vi "MiniCyc_Controller.vi"() -> ()   [LabVIEW 2024]
uses:
  <vilib>/Utility/file.llb/Write Delimited Spreadsheet (string).vi
panel:
  in  "Tab Control":T1(tab)
  in  "Tension Arc":dbl
  in  "Courant Arc":dbl
  in  "Réglage Arc :":enum32{"Item 0", "Item 1"}(radio)
  out "Tension effective Arc":dbl
  out "Courant effectif Arc":dbl
  in  "Courant Filament":dbl
  out "Courant effectif\nFilament":dbl
  in  "Débit Gaz m³/h":dbl(knob) scale=0.01..10.0 scale format="%#.6f"
  in  "Tension inflecteur":dbl min=0.0
  out "Tension I électrode 1":dbl
  out "Tension I électrode 2":dbl=-0.0
  out "Q2 Tension 2":dbl=-0.0
  in  "Tension quadrupole 2":dbl
  out "Q2 Tension 1":dbl
  out "Q1 Tension 2":dbl=-0.0
  in  "Tension quadrupole 1":dbl
  out "Q1 Tension 1":dbl
  in  "Tension Buncher":dbl
  out "Courant":bool=TRUE
  out "Débit Argon m³/h":dbl(knob) scale=0.0..10.0
  in  "Tension déflecteur":dbl min=0.0
  out "Tension D électrode 1":dbl
  out "Tension D électrode 2":dbl=-0.0
  in  "Tension Einzel":dbl
  in  "Tension Puller":dbl
  out "Tension effective\nEinzel":dbl
  out "Tension effective\nPuller":dbl
  out "Courant effectif\nBobine":dbl
  in  "Courant Bobine":dbl
  in  "Position\nPiston d'accord":dbl(knob) scale=0.01..10.0 scale format="%#.6f"
  out "Tension Crête":dbl
  out "Position effective\nPiston d'accord":dbl(slide) caption="Piston d'accord" scale=0.0..10.0
  in  "Amplificateur":dbl
  in  "Cible 1":enum32{"Item 0", "Item 1", "Radio Selection 3"}(radio)
  out "Courant Stripper1 Cible1":dbl
  out "Courant Stripper2 Cible1":dbl
  out "Courant Stripper3 Cible1":dbl
  in  "Rayon canne\nCible 1":dbl
  in  "Cible 2":enum32{"Item 0", "Item 1", "Radio Selection 3"}(radio)
  out "Courant Stripper1 Cible2":dbl
  out "Courant Stripper2 Cible2":dbl
  out "Courant Stripper3 Cible2":dbl
  in  "Rayon canne\nCible 2":dbl
  in  "Statut de la pompe":bool=TRUE
  out "Sonde 2 mbar":dbl(knob) scale=0.0..10.0
  out "Sonde 1 mbar":dbl(knob) scale=0.0..10.0
  out "Sonde 2 mbar":dbl(knob) scale=0.0..10.0
  out "Sonde 1 mbar":dbl(knob) scale=0.0..10.0
  out "Débit Eau\nBobine m³/h":dbl(knob) scale=0.0..10.0
  out "Débit Eau\nInflecteur m³/h":dbl(knob) scale=0.0..10.0
  out "Débit Eau\nDéflecteur m³/h":dbl(knob) scale=0.0..10.0
  out "Débit Eau\nLEBT m³/h":dbl(knob) scale=0.0..10.0
  out "Débit Eau\nSource m³/h":dbl(knob) scale=0.0..10.0
  out "Chemin du dossier":path
  in  "Limite de taille par fichiers":dbl=15.0
  in  "Activer l'enregistrement des données":bool=TRUE
  in  "Fréquence d'enregistrement des données":dbl=5.0
  # "KV"
  # "KV"
  # "mA"
  # "mA"
  # "µA"
  # "µA"
  # "KV"
  # "KV"
  # "KV"
  # "KV"
  # "KV"
  # "KV"
  # "KV"
  # "KV"
  # "KV"
  # "KV"
  # "KV"
  # "KV"
  # "KV"
  # "KV"
  # "KV"
  # "KV"
  # "KV"
  # "µA"
  # "µA"
  # "KV"
  # "µA"
  # "µA"
  # "µA"
  # "µA"
  # "µA"
  # "µA"
  # "Sec"
  # "Mb"
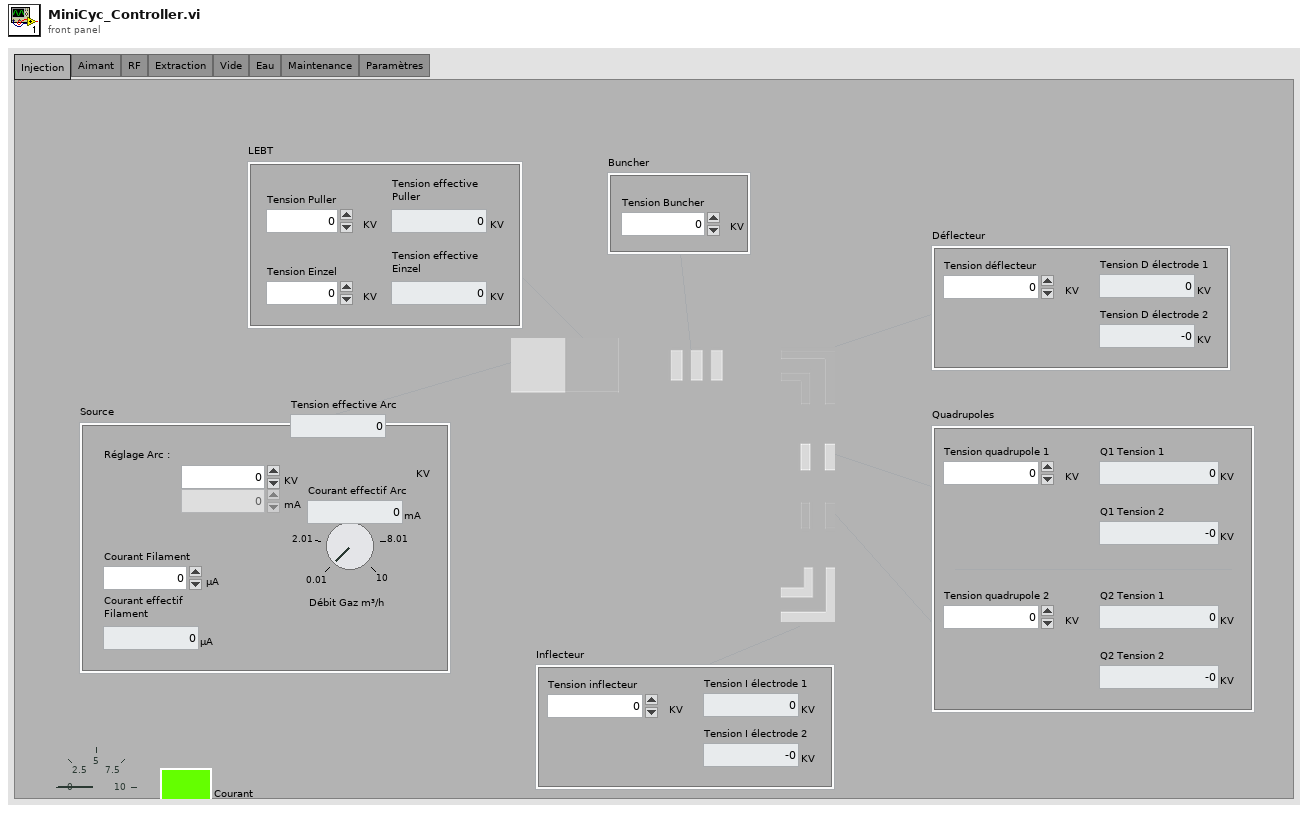
[diagram p1: front panel]
types:
  T1 = enum32{"Injection", "Aimant", "RF", "Extraction", "Vide", "Eau", "Maintenance", "Paramètres"}
  T2 = enum8{"Enabled", "Disabled", "Disabled and Grayed Out"}
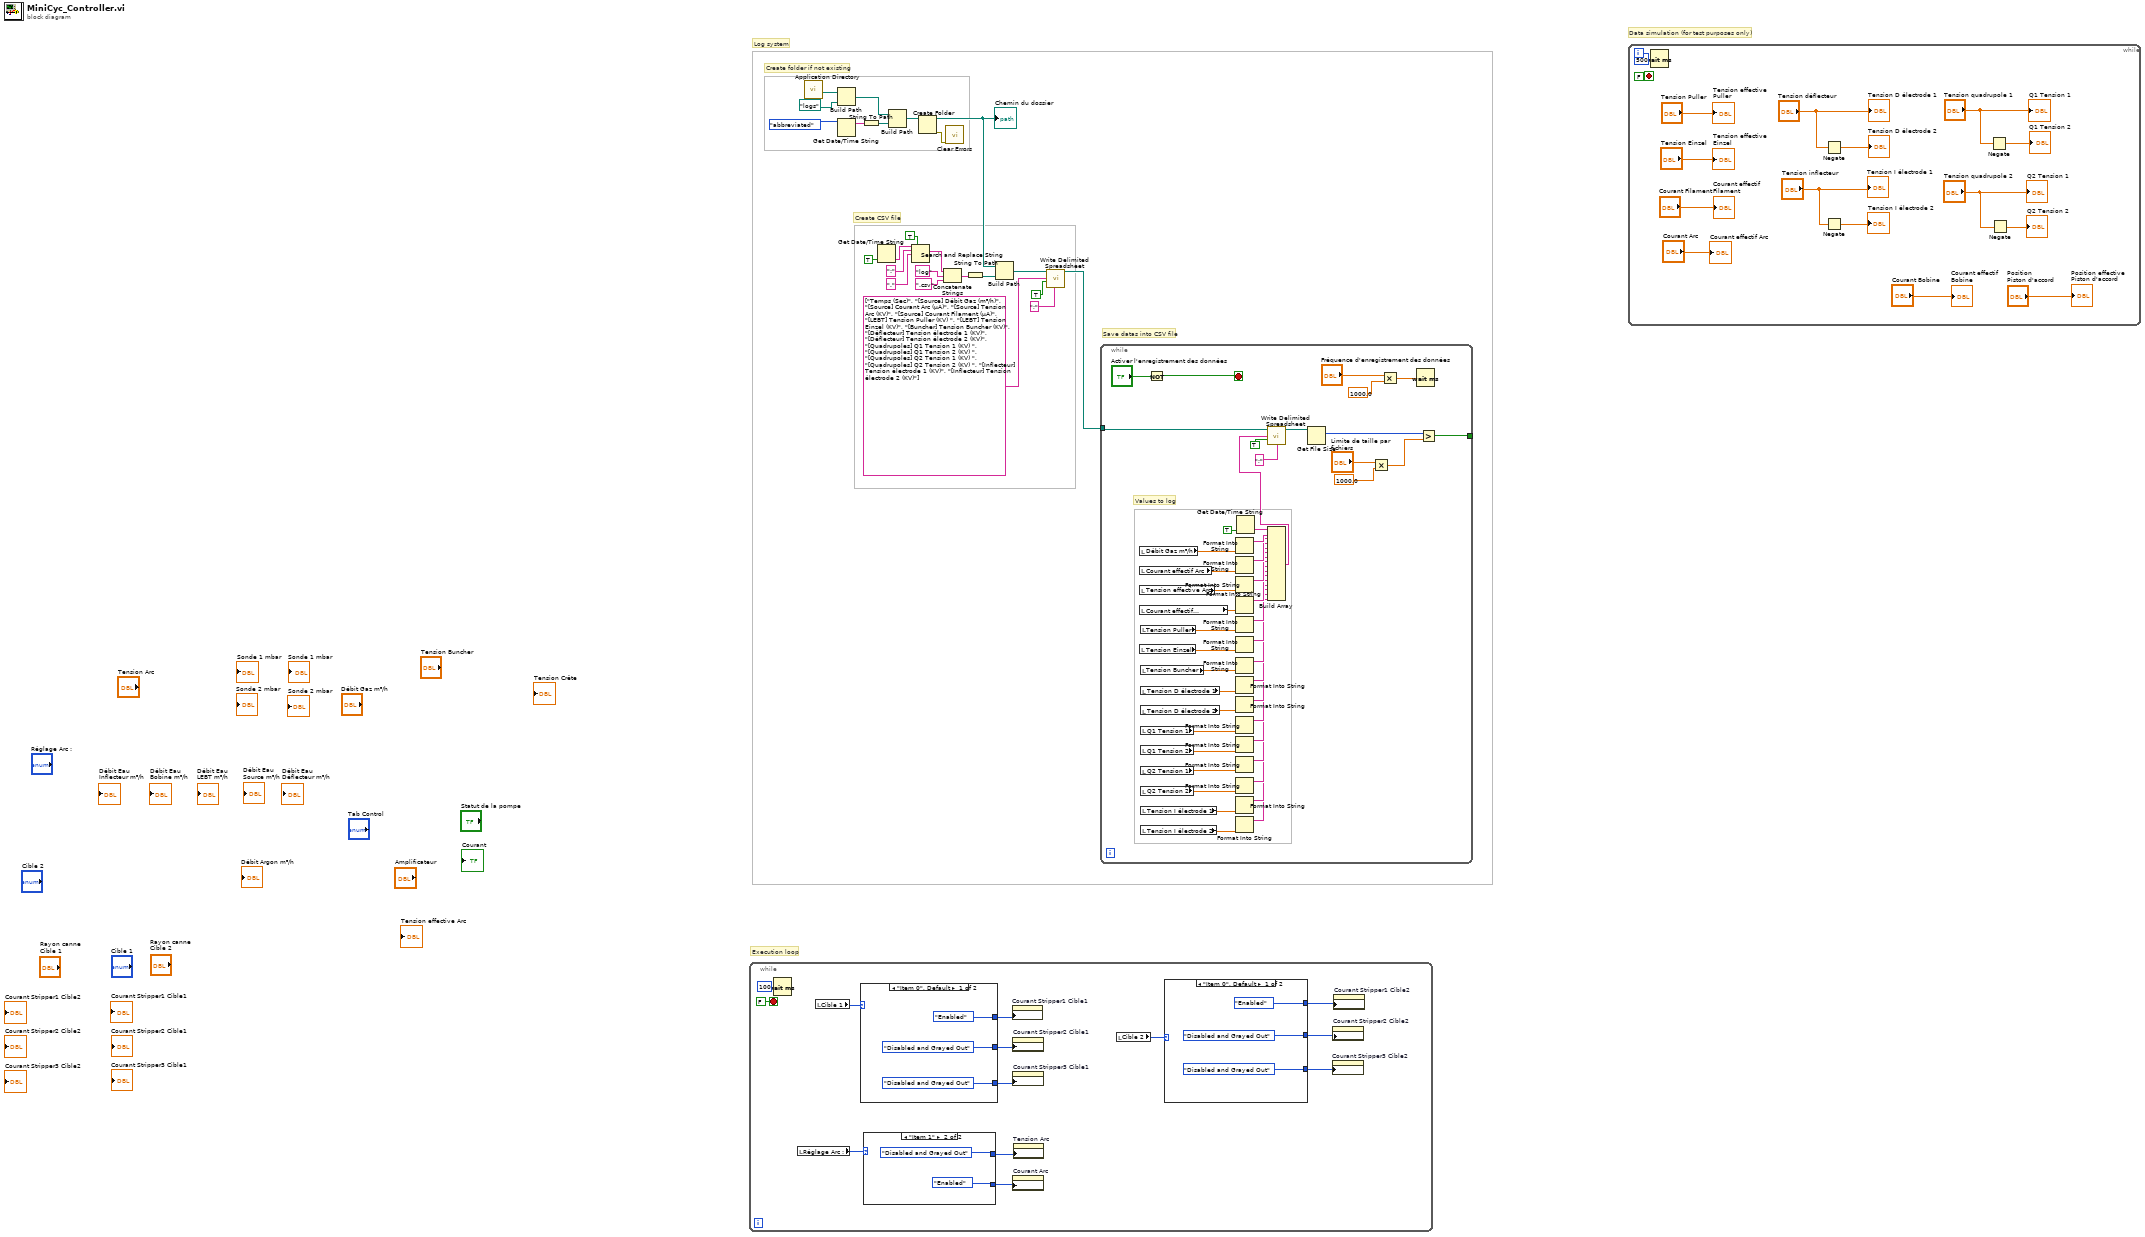
[diagram p0: block diagram]
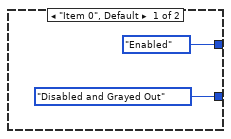
[diagram p2: hidden frame]
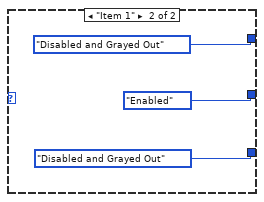
[diagram p3: hidden frame]
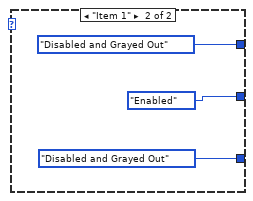
[diagram p4: hidden frame]
diagram:
  # "Execution loop"
  # "Log system"
  # "Data simulation (for test purposes only)"
  # "Save datas into CSV file"
  # "Create CSV file"
  # "Create folder if not existing"
  n1 = while {
    stop <- FALSE stop-if-true
    n2 = Wait (ms)(milliseconds to wait=u32 100) -> ()  [unwired: 1 out]
    n3 = local read "Réglage Arc :"() -> (w27:enum32{"Item 0", "Item 1"})
    n4 = local read "Cible 1"() -> (w32:enum32{"Item 0", "Item 1", "Radio Selection 3"})
    n5 = case shown="\"Item 0\", Default" w32 {
      tunnel: [T2."Disabled and Grayed Out" ("Disabled") T2."Disabled and Grayed Out" ("Disabled")] -> w33
      tunnel: [T2."Disabled and Grayed Out" ("Disabled") T2."Enabled" ("Disabled")] -> w34
      tunnel: [T2."Enabled" ("Disabled") T2."Disabled and Grayed Out" ("Disabled")] -> w35
      frame "Item 0", Default {
      }
      frame "Item 1" {
      }
    }
    n6 = case shown="\"Item 1\"" w27 {
      tunnel: [T2."Enabled" ("Disabled") T2."Disabled and Grayed Out" ("Disabled")] -> w26
      tunnel: [T2."Disabled and Grayed Out" ("Disabled") T2."Enabled" ("Disabled")] -> w25
      frame "Item 0", Default {
      }
      frame "Item 1" {
      }
    }
    n7 = property on="Courant Stripper1 Cible1" class="DigNum (strict)"("DisabledEnum"=w35) -> ()  [unwired: 2 in, 2 out]
    n8 = property on="Courant Stripper2 Cible1" class="DigNum (strict)"("DisabledEnum"=w34) -> ()  [unwired: 2 in, 2 out]
    n9 = property on="Courant Stripper3 Cible1" class="DigNum (strict)"("DisabledEnum"=w33) -> ()  [unwired: 2 in, 2 out]
    n10 = property on="Courant Arc" class="DigNum (strict)"("DisabledEnum"=w25) -> ()  [unwired: 2 in, 2 out]
    n11 = property on="Tension Arc" class="DigNum (strict)"("DisabledEnum"=w26) -> ()  [unwired: 2 in, 2 out]
    n12 = local read "Cible 2"() -> (w31:enum32{"Item 0", "Item 1", "Radio Selection 3"})
    n13 = case shown="\"Item 0\", Default" w31 {
      tunnel: [T2."Enabled" ("Disabled") T2."Disabled and Grayed Out" ("Disabled")] -> w30
      tunnel: [T2."Disabled and Grayed Out" ("Disabled") T2."Enabled" ("Disabled")] -> w29
      tunnel: [T2."Disabled and Grayed Out" ("Disabled") T2."Disabled and Grayed Out" ("Disabled")] -> w28
      frame "Item 0", Default {
      }
      frame "Item 1" {
      }
    }
    n14 = property on="Courant Stripper3 Cible2" class="DigNum (strict)"("DisabledEnum"=w28) -> ()  [unwired: 2 in, 2 out]
    n15 = property on="Courant Stripper2 Cible2" class="DigNum (strict)"("DisabledEnum"=w29) -> ()  [unwired: 2 in, 2 out]
    n16 = property on="Courant Stripper1 Cible2" class="DigNum (strict)"("DisabledEnum"=w30) -> ()  [unwired: 2 in, 2 out]
  }
  n17 = call <vilib>:"Application Directory.vi"() -> ("Application Directory"=w18:path)
  n18 = Build Path(base path=w18, name or relative path=path "logs" ("path (use dialog)")) -> (appended path=w16:path)
  n19 = Get Date/Time String(date format (0)=enum16{"short", "long", "abbreviated"}."abbreviated") -> (date string=w22:string)  [unwired: 2 in, 1 out]
  n20 = String To Path(string=w22) -> (path=w21:path)
  n21 = Get Date/Time String(want seconds? (F)=TRUE) -> (time string=w6:string)  [unwired: 2 in, 1 out]
  n22 = Build Path(base path=w16, name or relative path=w21) -> (appended path=w20:path)
  n23 = Search and Replace String(replace all?=TRUE ("replace all? (F)"), input string=w6, search string=":" ("replace string (\"\")"), replace string="." ("replace string (\"\")")) -> (result string=w7:string)  [unwired: 4 in, 3 out]
  n24 = Create Folder(path (use dialog)=w20) -> (created path=w14:path, error out=w24:errorcluster)  [unwired: 2 in, 1 out]
  "Chemin du dossier" <- w14
  n25 = Concatenate Strings(w7, "log" ("string"), ".csv" ("string")) -> (w12:string)
  n26 = call <vilib>:"Clear Errors.vi"("error in (no error)"=w24) -> ()  [unwired: 5 in, 2 out]
  n27 = String To Path(string=w12) -> (path=w15:path)
  n28 = Build Path(base path=w14, name or relative path=w15) -> (appended path=w10:path)
  n29 = call-poly <vilib>:"Write Delimited Spreadsheet.vi"("file path (dialog if empty)"=w10, "1D data"=string[] ["Temps (Sec)", "[Source] Débit Gaz (m³/h)", "[Source] Courant Arc (µA)", "[Source] Tension Arc (KV)", "[Source] Courant Filament (µA)", "[LEBT] Tension Puller (KV) ", "[LEBT] Tension Einzel (KV)", "[Buncher] Tension Buncher (KV)", "[Déflecteur] Tension électrode 1 (KV)", "[Déflecteur] Tension électrode 2 (KV)", "[Quadrupoles] Q1 Tension 1 (KV) ", "[Quadrupoles] Q1 Tension 2 (KV) ", "[Quadrupoles] Q2 Tension 1 (KV) ", "[Quadrupoles] Q2 Tension 2 (KV) ", "[Inflecteur] Tension électrode 1 (KV)", "[Inflecteur] Tension électrode 2 (KV)"] ("array"), "append to file? (new file:F)"=TRUE, "delimiter (\\t)"=";" ("delimiter (\\t)")) -> ("new file path (Not A Path if cancelled)"=w1:path)  [unwired: 10 in, 1 out]
  n30 = while {
    tunnel: w1 -> [w97]
    tunnel: [w92] -> _
    stop <- w87 stop-if-true
    # "Values to log"
    n31 = local read "Débit Gaz m³/h"() -> (w84:dbl)
    n32 = local read "Courant effectif Arc"() -> (w86:dbl)
    n33 = local read "Tension effective Arc"() -> (w79:dbl)
    n34 = local read "Courant effectif\nFilament"() -> (w77:dbl)
    n35 = local read "Tension Einzel"() -> (w75:dbl)
    n36 = local read "Tension Puller"() -> (w76:dbl)
    n37 = local read "Tension Buncher"() -> (w74:dbl)
    n38 = local read "Tension D électrode 1"() -> (w73:dbl)
    n39 = local read "Tension D électrode 2"() -> (w72:dbl)
    n40 = local read "Q1 Tension 1"() -> (w71:dbl)
    n41 = local read "Q1 Tension 2"() -> (w70:dbl)
    n42 = local read "Q2 Tension 1"() -> (w69:dbl)
    n43 = local read "Q2 Tension 2"() -> (w68:dbl)
    n44 = local read "Tension I électrode 1"() -> (w67:dbl)
    n45 = local read "Tension I électrode 2"() -> (w66:dbl)
    n46 = Not(x="Activer l'enregistrement des données") -> (.not. x?=w87:bool)
    n47 = Format Into String(w84) -> (resulting string=w81:string)  [unwired: 3 in, 1 out]
    n48 = Format Into String(w86) -> (resulting string=w80:string)  [unwired: 3 in, 1 out]
    n49 = Format Into String(w79) -> (resulting string=w78:string)  [unwired: 3 in, 1 out]
    n50 = Format Into String(w77) -> (resulting string=w65:string)  [unwired: 3 in, 1 out]
    n51 = Format Into String(w76) -> (resulting string=w64:string)  [unwired: 3 in, 1 out]
    n52 = Format Into String(w75) -> (resulting string=w63:string)  [unwired: 3 in, 1 out]
    n53 = Format Into String(w74) -> (resulting string=w62:string)  [unwired: 3 in, 1 out]
    n54 = Format Into String(w73) -> (resulting string=w61:string)  [unwired: 3 in, 1 out]
    n55 = Format Into String(w72) -> (resulting string=w60:string)  [unwired: 3 in, 1 out]
    n56 = Format Into String(w71) -> (resulting string=w59:string)  [unwired: 3 in, 1 out]
    n57 = Format Into String(w70) -> (resulting string=w58:string)  [unwired: 3 in, 1 out]
    n58 = Format Into String(w69) -> (resulting string=w57:string)  [unwired: 3 in, 1 out]
    n59 = Format Into String(w68) -> (resulting string=w56:string)  [unwired: 3 in, 1 out]
    n60 = Format Into String(w67) -> (resulting string=w55:string)  [unwired: 3 in, 1 out]
    n61 = Format Into String(w66) -> (resulting string=w54:string)  [unwired: 3 in, 1 out]
    n62 = Get Date/Time String(want seconds? (F)=TRUE) -> (time string=w85:string)  [unwired: 2 in, 1 out]
    n63 = Build Array(w85, w81, w80, w78, w65, w64, w63, w62, w61, w60, w59, w58, w57, w56, w55, w54) -> (w82:string[])
    n64 = call-poly <vilib>:"Write Delimited Spreadsheet.vi"("file path (dialog if empty)"=w97, "1D data"=w82, "append to file? (new file:F)"=TRUE, "delimiter (\\t)"=";" ("delimiter (\\t)")) -> ("new file path (Not A Path if cancelled)"=w94:path)  [unwired: 10 in, 1 out]
    n65 = Get File Size(file=w94) -> (size (in bytes)=w93:i64)  [unwired: 1 in, 2 out]
    n66 = Multiply(x="Limite de taille par fichiers", y=1000.0) -> (x*y=w90:dbl)
    n67 = Multiply(x="Fréquence d'enregistrement des données", y=1000.0) -> (x*y=w98:dbl)
    n68 = Wait (ms)(milliseconds to wait=w98) -> ()  [unwired: 1 out]
    n69 = Greater?(x=w93, y=w90) -> (0:w92:bool)
  }
  n70 = while {
    stop <- FALSE stop-if-true
    n71 = Wait (ms)(milliseconds to wait=u32 500) -> ()  [unwired: 1 out]
    n72 = Negate(x="Tension déflecteur") -> (-x=→"Tension D électrode 2":dbl)
    n73 = Negate(x="Tension inflecteur") -> (-x=→"Tension I électrode 2":dbl)
    n74 = Negate(x="Tension quadrupole 1") -> (-x=→"Q1 Tension 2":dbl)
    n75 = Negate(x="Tension quadrupole 2") -> (-x=→"Q2 Tension 2":dbl)
    "Courant effectif Arc" <- "Courant Arc"
    "Tension effective\nPuller" <- "Tension Puller"
    "Tension effective\nEinzel" <- "Tension Einzel"
    "Courant effectif\nFilament" <- "Courant Filament"
    "Tension D électrode 1" <- "Tension déflecteur"
    "Tension I électrode 1" <- "Tension inflecteur"
    "Q1 Tension 1" <- "Tension quadrupole 1"
    "Q2 Tension 1" <- "Tension quadrupole 2"
    "Courant effectif\nBobine" <- "Courant Bobine"
    "Position effective\nPiston d'accord" <- "Position\nPiston d'accord"
  }
